vi "Math Lookup.vi"() -> ()   [LabVIEW 2014]
doc: "This example shows how to apply a lookup table to an image. Lookup table (LUT) transformations are basic mathematical functions that can be used to improve the contrast and brightness of an image by modifying the intensity dynamics of regions with poor contrast. The LUT can also be used to highlight details in areas containing significant information. In NI Vision, apart from the predefined functions that can be used through the IMAQ MathLookup VI, you can also apply your own lookup tables using the IMAQ UserLookup VI."
uses:
  <vilib>/vision/NI_Vision_Development_Module.lvlib
panel:
  out "Hist-Dst":T1(graph)
  out "H-Src":T1(graph)
  in  "Stop Button":bool
  in  "Operator":u16(ring)=3 items=["Linear", "Log", "Exp", "Square", "Square root", "Power X", "Power 1/X"]
  in  "X for Power X, 1/X":sgl=1.5 min=0 format="%_3g"
  out "LUT Image":T2(plugin-control) caption="Lut Image"
  out "Image Source":T2(plugin-control)
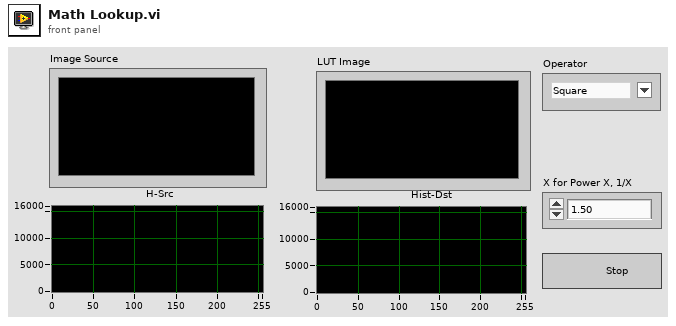
[diagram p1: front panel]
types:
  T1 = cluster{"Starting Value":sgl, "Incremental Value":sgl, "Histogram":u32[]}
  T2 = typedef "IMAQ Image.ctl" = refnum<image>
  T3 = typedef "Image Type" = u32
  T4 = cluster{"X for Power X, 1/X":sgl, "Operator":u16}
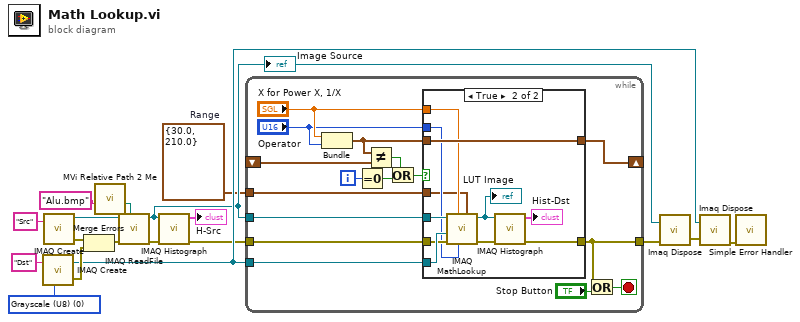
[diagram p0: block diagram]
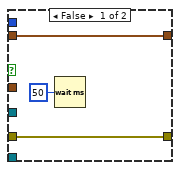
[diagram p2: hidden frame]
diagram:
  w1 = cluster{"Minimum":sgl, "Maximum":sgl} {"Minimum"=30.0, "Maximum"=210.0}  # Range
  w14 = T3 0 items=["Grayscale (U8)", "Grayscale (I16)", "Grayscale (SGL)", "Complex (CSG)", "RGB (U32)", "HSL (U32)", "RGB (U64)", "Grayscale (U16)"] ("Image Type")
  n1 = call "IMAQ Create"("Image Name"="Dst", "Image Type"=w14) -> ("New Image"=w9:T2, "error out"=w13:errorcluster)  [unwired: 3 in]
  n2 = call "IMAQ Create"("Image Name"="Src") -> ("New Image"=w17:T2, "error out"=w11:errorcluster)  [unwired: 4 in]
  n3 = Merge Errors(w11, w13) -> (w12:errorcluster)
  n4 = call "MVi Relative Path 2 Me.vi"("Relative Path"="Alu.bmp" ("name or relative path")) -> ("Appended Dir"=w6:path)  [unwired: 5 in, 1 out]
  n5 = call "IMAQ ReadFile"("File Path"=w6, "error in (no error)"=w12, "Image"=w17) -> ("error out"=w5:errorcluster, "Image Out"=w4:T2)  [unwired: 4 in, 3 out]
  "Image Source" <- w4
  n6 = call "IMAQ Histograph"("error in (no error)"=w5, "Image"=w4) -> ("error out"=w3:errorcluster, "Histogram Graph"=→"H-Src":T1)  [unwired: 6 in, 2 out]
  n7 = while {
    tunnel: w3 -> [w34]
    tunnel: w4 -> [w33]
    tunnel: w9 -> [w32]
    shift-right: [w31] -> _
    shift-left: _ -> [w30]
    tunnel: [w24] -> w10
    tunnel: w1 -> [w19]
    i -> [w29]
    stop <- w23 stop-if-true
    n8 = Bundle("X for Power X, 1/X"="X for Power X, 1/X", "Operator"="Operator") -> (w20:T4)  [unwired: 1 in]
    n9 = Equal To 0?(x=w29) -> (x = 0?=w27:bool)
    n10 = Not Equal?(x=w20, y=w30) -> (x != y?=w28:bool)
    n11 = Or(x=w28, y=w27) -> (x .or. y?=w26:bool)
    n12 = case shown="True" w26 {
      tunnel: w34 -> [w37 w46]
      tunnel: w33 -> [_ w45]
      tunnel: w20 -> [w36 w48]
      tunnel: w32 -> [_ w47]
      tunnel: [w36 w48] -> w31
      tunnel: [w37 w41] -> w24
      tunnel: "X for Power X, 1/X" -> [_ w44]
      tunnel: "Operator" -> [_ w43]
      tunnel: w19 -> [_ w38]
      frame False {
        n13 = Wait (ms)(milliseconds to wait=u32 50) -> ()  [unwired: 1 out]
      }
      frame True {
        n14 = call "IMAQ MathLookup"("Range"=w38, "Operator"=w43, "X Value"=w44, "error in (no error)"=w46, "Image Dst"=w47, "Image Src"=w45) -> ("error out"=w42:errorcluster, "Image Dst Out"=w40:T2)  [unwired: 4 in]
        "LUT Image" <- w40
        n15 = call "IMAQ Histograph"("error in (no error)"=w42, "Image"=w40) -> ("error out"=w41:errorcluster, "Histogram Graph"=→"Hist-Dst":T1)  [unwired: 6 in, 2 out]
      }
    }
    n16 = Or(x=w24, y="Stop Button") -> (x .or. y?=w23:bool)
  }
  n17 = call "Imaq Dispose"("Image"=w4, "error in (no error)"=w10) -> ("error out"=w8:errorcluster)  [unwired: 4 in]
  n18 = call "Imaq Dispose"("Image"=w9, "error in (no error)"=w8) -> ("error out"=w16:errorcluster)  [unwired: 4 in]
  n19 = call <vilib>:"Simple Error Handler.vi"("error in (no error)"=w16) -> ()  [unwired: 4 in, 5 out]
